vi "Maximum Corr coeff.vi"() -> (5 "Plug in titles":string[](array[string]), 7 "Plug in values":string[](array[string]))   [LabVIEW 2015]
uses:
  <vilib>/Analysis/3filter.llb/Filter Passband Type.ctl
  Globals/Meas_global.vi
  <vilib>/Analysis/3filter.llb/Zero Phase Filter (Cascade, DBL).vi
  <vilib>/Analysis/NI_AALBase.lvlib
panel:
  in  "Minimum Correlation Coefficient\nto give time lag for":dbl=0.1
  in  "Time Trace":bool=TRUE
  in  "Wind turbine location\n(Applicable only if \nInput own variables? is OFF)":dbl=10000.0
  out "XY Graph 3":cluster{"Time (ms)":dbl[], "Eng Values":dbl[]}[](graph)
  out "Error":i32
  in  "Filter 2nd Instrument data?":bool
  in  "Freq Cutoff Inst 2":dbl=100.0
  in  "Freq Cutoff Inst 1":dbl=100.0
  in  "Filter 1st Instrument Data?":bool
  in  "Start point(s)":dbl
  in  "Time step (s)":dbl=0.05
  in  "Input own variables?":bool=TRUE
  out "Start point":dbl
  out "XY Graph 2":cluster{dbl[], dbl[]}(graph)
  out "Time step":dbl
  in  "Number of estimates":i32=20
  out "Time Trace":cluster{"Time (ms)":dbl[], "Eng Values":dbl[]}[](graph)
  in  "Instrumnt 2":i32=1
  in  "Instrument 1":i32
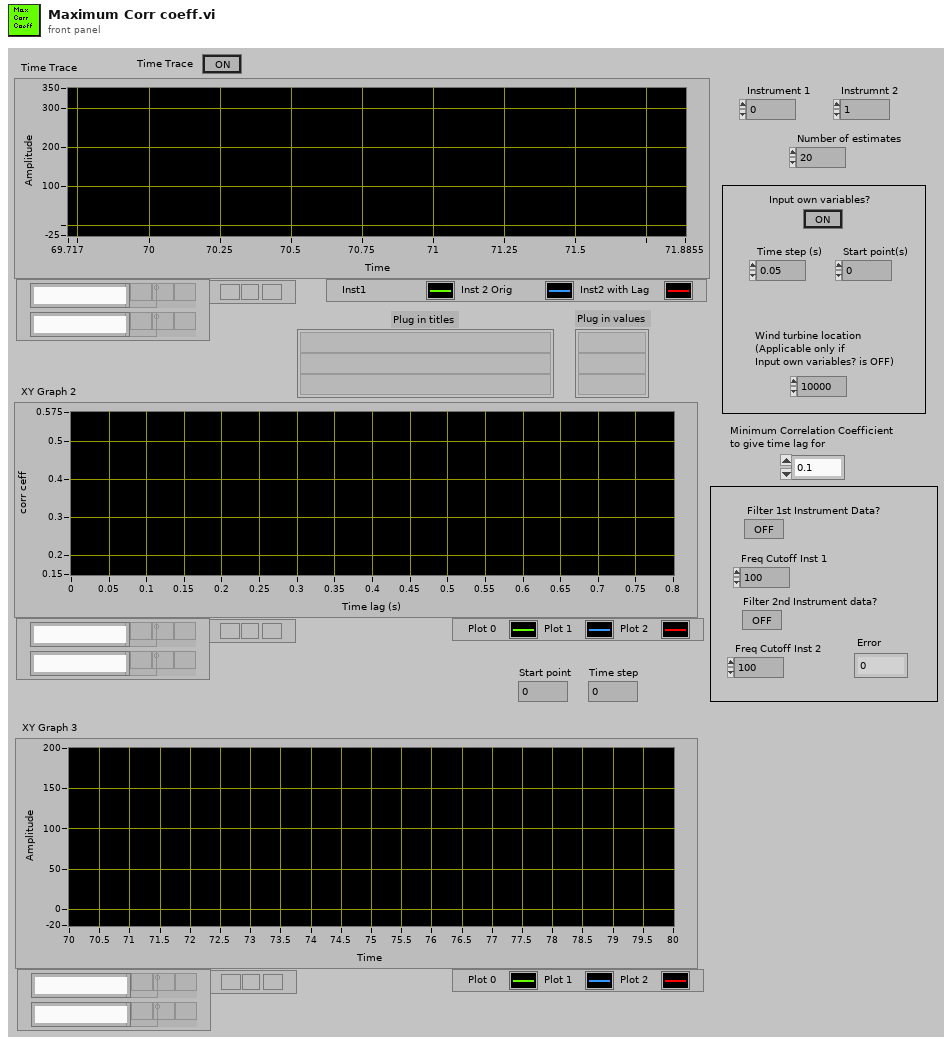
[diagram p1: front panel]
types:
  T1 = typedef "Time_Trace_Cluster.ctl" = cluster{"Weighting":dbl[], "Time (s)":dbl[], "Voltage":dbl[], "Eng Values":dbl[]}
  T2 = typedef "Analysis_info_cluster.ctl" = cluster{"Colour":u32, "Inst type":T3, "Inst name":string, "Symbol":string, "Code name":string, "Extra Info":string, "Inst Array":T4, "Extra Titles":string[], "Extra Values":string[], "U":dbl, "u^2":dbl, "u^3":dbl, "u^4":dbl, "Skew_u":dbl, "Kurt_u":dbl, "Sd Error in Mean":dbl, "% u'/U":dbl, "X":dbl, "Y":dbl, "Z":dbl, "Timescale integral to 25%":dbl, "Sd Error in Variance":dbl, "Calib File":path, "Calib Constants":dbl[], "Output Position":bool, "Full Stats":bool, "Av Sampling Rate":dbl, "Av No of Samples":dbl, "Total Meas Time (s)":dbl, "ADAM Ch Name":string, "Max value":dbl, "Min value":dbl}
  T3 = typedef "Inst_type.ctl" = enum16{"Propeller anemometer", "Raw voltage", "Pressure Transducer", "Pitot-static tube", "Preston tube", "Hot wire", "Cross wire 1", "Cross wire 2", "Generic Linear", "Generic Polynomial", "Generic BackPoly", "Fast FID", "Thermocouple", "Cold wire", "Pulsed Wire", "LDA Vel", "LDA Tran time", "LDA Arr time", "Microphone"}
  T4 = typedef "Instrument_Array.ctl" = enum16{"PWA", "LDA", "Analogue"}
  T5 = typedef "NI_AALBase.lvlib/Filter Passband Type.ctl" = enum32{"Lowpass", "Highpass", "Bandpass", "Bandstop"}
  T6 = cluster{"filter structure":enum32{"IIR 2nd Order", "IIR 4th Order"}, "Reverse Coefficients":dbl[], "Forward Coefficients":dbl[]}
  T7 = typedef "Correlation_cluster1.ctl" = cluster{"U inst":string, "uw":dbl, "u^2w":dbl, "uw^2":dbl, "uw/u'w'":dbl, "W inst":string, "uw^3":dbl, "u^3w":dbl, "u^2w^2":dbl, "Index U":i32, "Index W":i32}
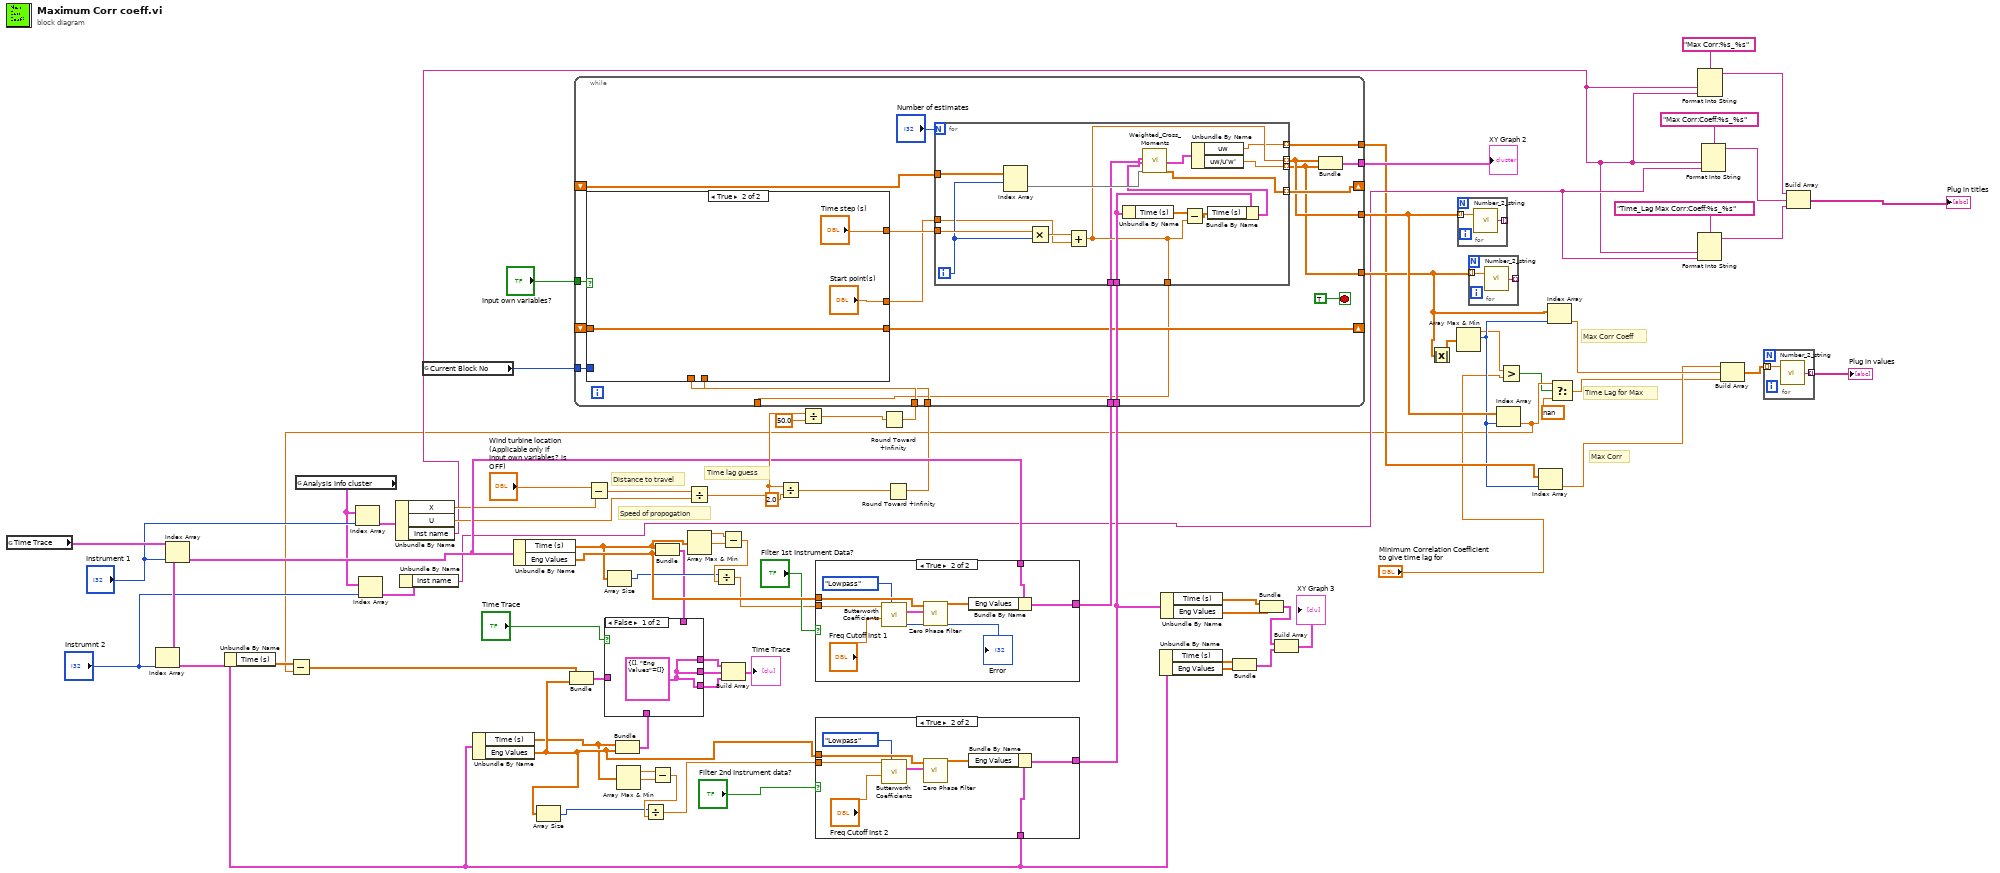
[diagram p0: block diagram]
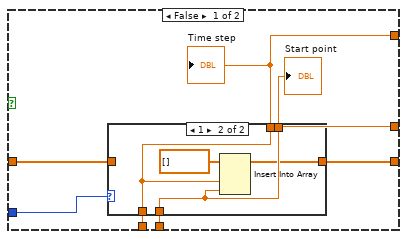
[diagram p5: hidden frame]
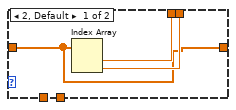
[diagram p6: hidden frame]
diagram:
  # "Max Corr"
  # "Time Lag for Max"
  # "Max Corr Coeff"
  # "Speed of propogation"
  # "Distance to travel"
  # "Time lag guess"
  n1 = global read "Meas_global.vi" "Time Trace"() -> (w80:T1[])
  n2 = Index Array(array=w80, index="Instrumnt 2") -> (element=w21:T1)
  n3 = Index Array(array=w80, index="Instrument 1") -> (element=w60:T1)
  n4 = Unbundle By Name(w21) -> ("Time (s)"=w79:dbl[])
  n5 = global read "Meas_global.vi" "Analysis Info cluster"() -> (w28:T2[])
  n6 = Index Array(array=w28, index="Instrument 1") -> (element=w41:T2)
  n7 = Index Array(array=w28, index="Instrumnt 2") -> (element=w29:T2)
  n8 = Unbundle By Name(w41) -> ("X"=w40:dbl, "U"=w39:dbl, "Inst name"=w9:string)
  n9 = Unbundle By Name(w29) -> ("Inst name"=w23:string)
  n10 = global read "Meas_global.vi" "Current Block No"() -> (w74:i32)
  n11 = Unbundle By Name(w21) -> ("Time (s)"=w44:dbl[], "Eng Values"=w61:dbl[])
  n12 = Unbundle By Name(w60) -> ("Time (s)"=w55:dbl[], "Eng Values"=w71:dbl[])
  n13 = Array Size(array=w61) -> (size(s)=w45:i32)
  n14 = Subtract(x="Wind turbine location\n(Applicable only if \nInput own variables? is OFF)", y=w40) -> (x-y=w38:dbl)
  n15 = Array Size(array=w55) -> (size(s)=w51:i32)
  n16 = Bundle("Time (s)"=w44, "Eng Values"=w61) -> (w15:cluster{"Time (s)":dbl[], "Eng Values":dbl[]})  [unwired: 1 in]
  n17 = Array Max & Min(array=w44) -> (max value=w47:dbl, min value=w48:dbl)  [unwired: 2 out]
  n18 = Subtract(x=w47, y=w48) -> (x-y=w46:dbl)
  n19 = Divide(x=w45, y=w46) -> (x/y=w49:dbl)
  n20 = Bundle("Time (s)"=w55, "Eng Values"=w71) -> (w18:cluster{"Time (s)":dbl[], "Eng Values":dbl[]})  [unwired: 1 in]
  n21 = Divide(x=w38, y=w39) -> (x/y=w76:dbl)
  n22 = Array Max & Min(array=w55) -> (max value=w54:dbl, min value=w53:dbl)  [unwired: 2 out]
  n23 = Subtract(x=w54, y=w53) -> (x-y=w52:dbl)
  n24 = Divide(x=w51, y=w52) -> (x/y=w50:dbl)
  n25 = Divide(x=w76, y=2.0) -> (x/y=w36:dbl)
  n26 = Divide(x=w76, y=50.0) -> (x/y=w35:dbl)
  n27 = case shown="True" "Filter 1st Instrument Data?" {
    tunnel: w71 -> [_ w90]
    tunnel: w50 -> [_ w89]
    tunnel: w60 -> [w82 w87]
    tunnel: [w82 w86] -> w70
    frame False {
    }
    frame True {
      n28 = call <vilib>:"Butterworth Coefficients.vi"("filter type"=Filter_Passband_Type."Lowpass", "low cutoff freq: fl"="Freq Cutoff Inst 1", "sampling freq: fs"=w89) -> ("error"=→"Error":i32, "IIR Filter Cluster"=w91:T6)  [unwired: 7 in]
      n29 = call-poly <vilib>:"Zero Phase Filter.vi"("IIR Filter Cluster"=w91, "X"=w90) -> ("Filtered X"=w88:dbl[])  [unwired: 8 in, 1 out]
      n30 = Bundle By Name(cluster=w87, "Eng Values"=w88) -> (w86:T1)
    }
  }
  n31 = case shown="True" "Filter 2nd Instrument data?" {
    tunnel: w61 -> [_ w99]
    tunnel: w49 -> [_ w98]
    tunnel: [w92 w96] -> w59
    tunnel: w21 -> [w92 w94]
    frame False {
    }
    frame True {
      n32 = call <vilib>:"Butterworth Coefficients.vi"("filter type"=Filter_Passband_Type."Lowpass", "low cutoff freq: fl"="Freq Cutoff Inst 2", "sampling freq: fs"=w98) -> ("IIR Filter Cluster"=w100:T6)  [unwired: 7 in, 1 out]
      n33 = call-poly <vilib>:"Zero Phase Filter.vi"("IIR Filter Cluster"=w100, "X"=w99) -> ("Filtered X"=w97:dbl[])  [unwired: 8 in, 1 out]
      n34 = Bundle By Name(cluster=w94, "Eng Values"=w97) -> (w96:T1)
    }
  }
  n35 = Round Toward +Infinity(x=w35) -> (ceil(x): smallest int >= x=w34:dbl)
  n36 = Round Toward +Infinity(x=w36) -> (ceil(x): smallest int >= x=w37:dbl)
  n37 = while {
    tunnel: w70 -> [w119]
    tunnel: w59 -> [w118]
    shift-right: [w116] -> _
    shift-left: _ -> [w115]
    tunnel: [w114] -> w78
    tunnel: [w112] -> w72
    tunnel: [w105] -> w56
    tunnel: w34 -> [w110]
    tunnel: w74 -> [w111]
    tunnel: w37 -> [w109]
    shift-right: [w108] -> _
    shift-left: _ -> [w107]
    tunnel: "Input own variables?" -> [w104]
    tunnel: [w102] -> _
    tunnel: [w101] -> w12
    stop <- TRUE stop-if-true
    n38 = case shown="True" w104 {
      tunnel: w111 -> [w126 _]
      tunnel: w110 -> [w125 _]
      tunnel: w109 -> [w124 _]
      tunnel: [w123 w134] -> w108
      tunnel: w107 -> [w122 w134]
      tunnel: [w121 "Start point(s)"] -> w103
      tunnel: [w120 "Time step (s)"] -> w106
      frame False {
        n39 = case shown="1" w126 {
          tunnel: w125 -> [_ w132]
          tunnel: [w129 w132] -> w120
          tunnel: [w128 w133] -> w121
          tunnel: w124 -> [_ w133]
          tunnel: [w127 w131] -> w123
          tunnel: w122 -> [w127 _]
          frame 2, Default {
            n40 = Index Array(array=w127) -> (element #1=w129:dbl, element #2=w128:dbl)  [unwired: 2 in]
          }
          frame 1 {
            n41 = Insert Into Array(array=dbl[] [], new element #1=w132, new element #2=w133) -> (w131:dbl[])  [unwired: 1 in]
          }
        }
        "Time step" <- w120
        "Start point" <- w121
      }
      frame True {
      }
    }
    n42 = for {
      N: "Number of estimates" -> [_]
      tunnel: w119 -> [w139]
      tunnel: w118 -> [w144]
      tunnel: w106 -> [w152]
      tunnel: [w150] -> w116 mode=indexing
      tunnel: w115 -> [w149]
      tunnel: [w140] -> w112 mode=indexing
      tunnel: [w147] -> w105 mode=indexing
      tunnel: w103 -> [w141]
      tunnel: [w140] -> w102
      tunnel: [w137] -> w101 mode=indexing
      i -> [w143]
      n43 = Index Array(array=w149, index (row)=w143) -> (element=w151:dbl[])  [unwired: 1 in]
      n44 = Multiply(x=w152, y=w143) -> (x*y=w142:dbl)
      n45 = Add(x=w142, y=w141) -> (x+y=w140:dbl)
      n46 = Unbundle By Name(w144) -> ("Time (s)"=w146:dbl[])
      n47 = Subtract(x=w146, y=w140) -> (x-y=w145:dbl[])
      n48 = Bundle By Name(cluster=w144, "Time (s)"=w145) -> (w138:T1)
      n49 = call "Weighted_Cross_Moments.vi"("Time Cluster 1"=w139, "Time Cluster 2"=w138, "Shift in"=w151) -> ("output cluster"=w148:T7, "Shift out"=w150:dbl[])  [unwired: 15 in]
      n50 = Unbundle By Name(w148) -> ("uw"=w137:dbl, "uw/u'w'"=w147:dbl)
    }
    n51 = Bundle(w112, w105) -> (w114:cluster{dbl[], dbl[]})  [unwired: 1 in]
  }
  "XY Graph 2" <- w78
  n52 = Unbundle By Name(w21) -> ("Time (s)"=w64:dbl[], "Eng Values"=w63:dbl[])
  n53 = Unbundle By Name(w59) -> ("Time (s)"=w66:dbl[], "Eng Values"=w65:dbl[])
  n54 = Bundle("Time (s)"=w64, "Eng Values"=w63) -> (w58:cluster{"Time (s)":dbl[], "Eng Values":dbl[]})  [unwired: 1 in]
  n55 = Bundle("Time (s)"=w66, "Eng Values"=w65) -> (w57:cluster{"Time (s)":dbl[], "Eng Values":dbl[]})  [unwired: 1 in]
  n56 = Build Array(w57, w58) -> (→"XY Graph 3":cluster{"Time (s)":dbl[], "Eng Values":dbl[]}[])
  n57 = Absolute Value(x=w56) -> (abs(x)=w67:dbl[])
  n58 = Array Max & Min(array=w67) -> (max value=w6:dbl, max index (indices)=w11:i32)  [unwired: 2 out]
  n59 = for {
    tunnel: w72 -> [w153] mode=indexing
    tunnel: [w154] -> _ mode=indexing
    n60 = call "Number_2_string.vi"("number"=w153) -> ("String"=w154:string)  [unwired: 1 in]
  }
  n61 = for {
    tunnel: w56 -> [w155] mode=indexing
    tunnel: [w156] -> _ mode=indexing
    n62 = call "Number_2_string.vi"("number"=w155) -> ("String"=w156:string)  [unwired: 1 in]
  }
  n63 = Index Array(array=w72, index=w11) -> (element=w4:dbl)
  n64 = Subtract(x=w79, y=w4) -> (x-y=w20:dbl[])
  n65 = Bundle(w20, "Eng Values"=w61) -> (w14:cluster{dbl[], "Eng Values":dbl[]})  [unwired: 1 in]
  n66 = case shown="False" "Time Trace" {
    tunnel: w18 -> [_ w160]
    tunnel: [w157 w160] -> w17
    tunnel: [w157 w159] -> w16
    tunnel: w15 -> [_ w159]
    tunnel: w14 -> [_ w158]
    tunnel: [w157 w158] -> w13
    frame False {
      w157 = cluster{dbl[], "Eng Values":dbl[]} {[], "Eng Values"=[]}
    }
    frame True {
    }
  }
  n67 = Build Array(w17, w16, w13) -> (→"Time Trace":cluster{"Time (s)":dbl[], "Eng Values":dbl[]}[])
  n68 = Greater?(x=w6, y="Minimum Correlation Coefficient\nto give time lag for") -> (0:w3:bool)
  n69 = Index Array(array=w12, index=w11) -> (element=w7:dbl)
  n70 = Index Array(array=w56, index=w11) -> (element=w31:dbl)
  n71 = Select(t=w4, s=w3, f=nan) -> (s? t:f=w1:dbl)
  n72 = Format Into String(format string="Time_Lag Max Corr:Coeff:%s_%s", w9, w23) -> (resulting string=w22:string)  [unwired: 2 in, 1 out]
  n73 = Format Into String(format string="Max Corr:%s_%s", w9, w9) -> (resulting string=w8:string)  [unwired: 2 in, 1 out]
  n74 = Format Into String(format string="Max Corr:Coeff:%s_%s", w9, w23) -> (resulting string=w25:string)  [unwired: 2 in, 1 out]
  n75 = Build Array(w7, w31, w1) -> (w33:dbl[])
  n76 = for {
    tunnel: w33 -> [w161] mode=indexing
    tunnel: [w162] -> w32 mode=indexing
    n77 = call "Number_2_string.vi"("number"=w161) -> ("String"=w162:string)  [unwired: 1 in]
  }
  "Plug in values" <- w32
  n78 = Build Array(w8, w25, w22) -> (→"Plug in titles":string[])
